vi "ramping waveform.vi"(6 "mode":u16(ring) items=["unidirection", "bidirection"], 8 "points in t2":dbl=500.0, 9 "points in t1":dbl=500.0, 10 "p2":dbl=10000.0, 11 "p1":dbl=10000.0) -> (3 "array":dbl[](array[numeric]))   [LabVIEW 2015]
panel:
  out "d":dbl=10000.0
  out "c":dbl=10000.0
  out "Waveform Graph":dbl[](graph)
  out "b":dbl=10000.0
  out "a":dbl=10000.0
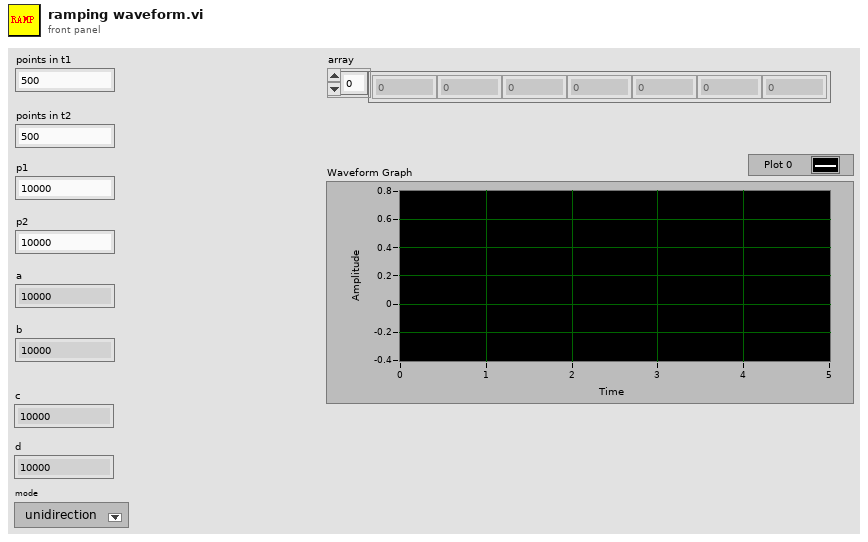
[diagram p1: front panel]
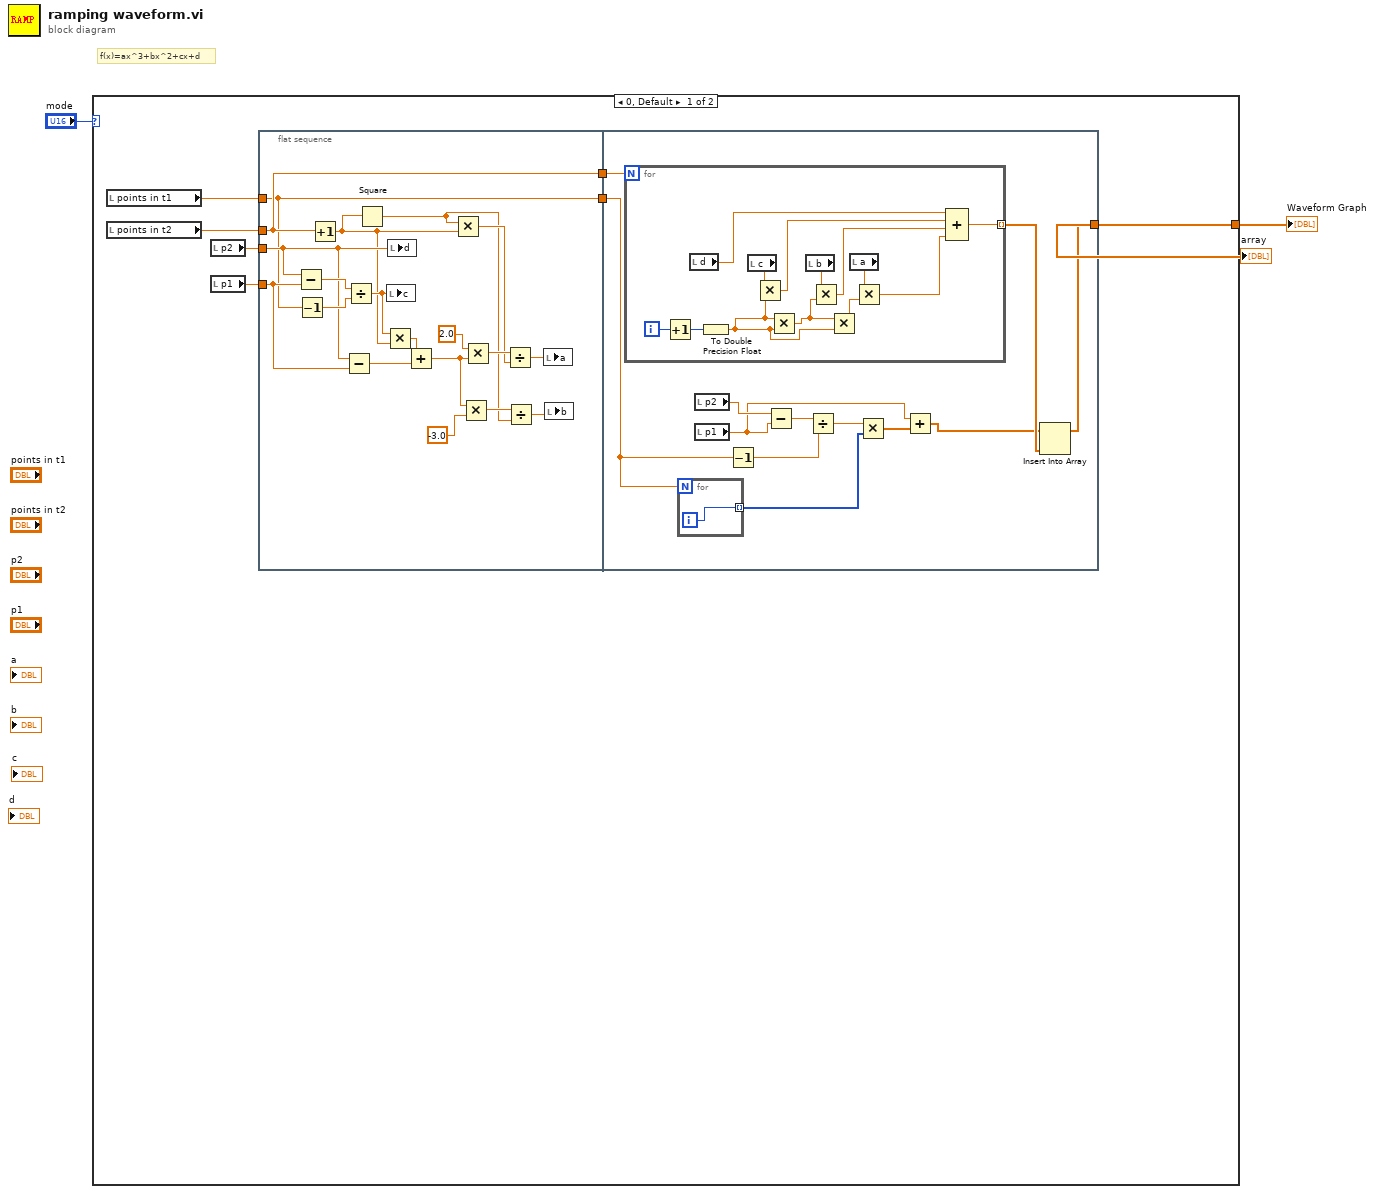
[diagram p0: block diagram]
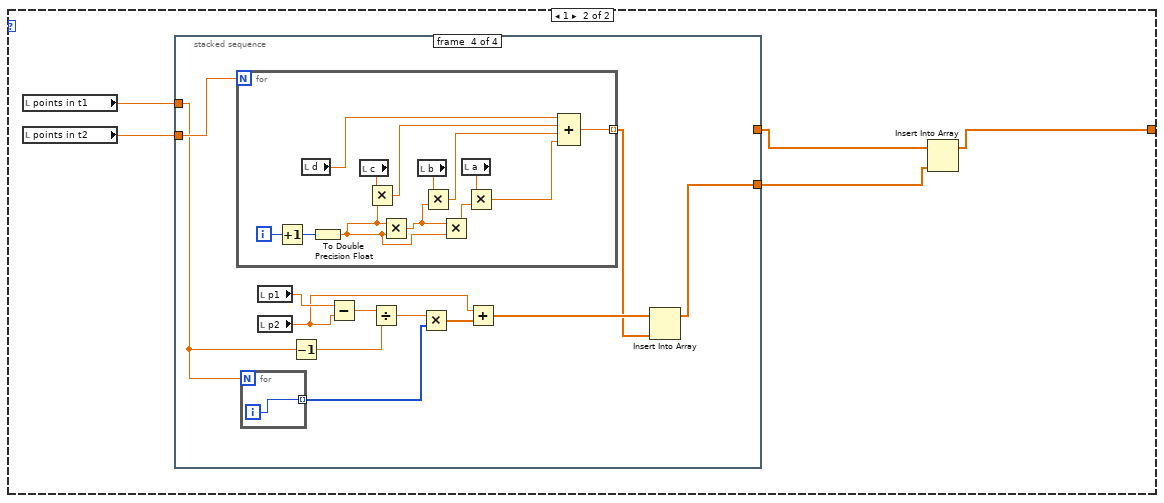
[diagram p2: hidden frame]
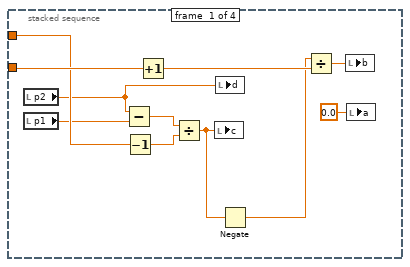
[diagram p3: hidden frame]
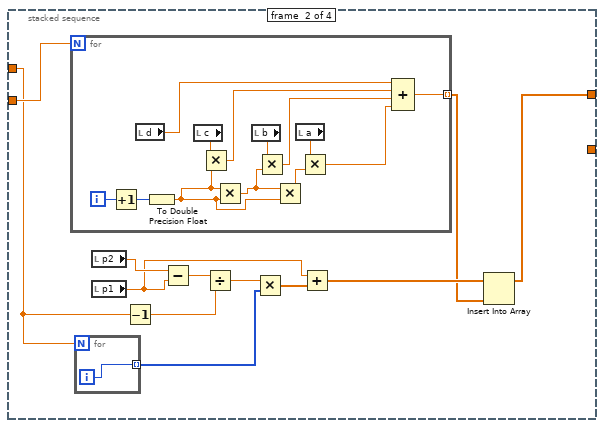
[diagram p4: hidden frame]
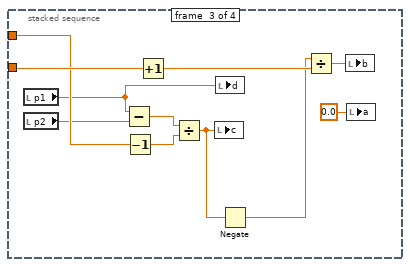
[diagram p5: hidden frame]
diagram:
  # "f(x)=ax^3+bx^2+cx+d"
  n1 = case shown="0, Default" "mode" {
    tunnel: [w9 w55] -> w1
    frame 0, Default {
      n2 = local read "points in t1"() -> (w5:dbl)
      n3 = local read "points in t2"() -> (w6:dbl)
      n4 = local read "p2"() -> (w7:dbl)
      n5 = local read "p1"() -> (w8:dbl)
      n6 = flat-sequence {
        tunnel: w6 -> [w24]
        tunnel: w7 -> [w23]
        tunnel: w8 -> [w22]
        tunnel: w5 -> [w10]
        tunnel: [w24] -> w4
        tunnel: [w10] -> w3
        tunnel: [w39] -> w9
        tunnel: w4 -> [w40]
        tunnel: w3 -> [w29]
        frame #0 {
          n7 = Subtract(x=w23, y=w22) -> (x-y=w28:dbl)
          n8 = Decrement(x=w10) -> (x-1=w27:dbl)
          n9 = Increment(x=w24) -> (x+1=w12:dbl)
          n10 = Subtract(x=w23, y=w22) -> (x-y=w20:dbl)
          n11 = Divide(x=w28, y=w27) -> (x/y=w25:dbl)
          n12 = Square(x=w12) -> (x^2=w11:dbl)
          n13 = Multiply(x=w25, y=w12) -> (x*y=w21:dbl)
          n14 = local write "c"(w25) -> ()
          n15 = local write "d"(w23) -> ()
          n16 = Add(x=w21, y=w20) -> (x+y=w16:dbl)
          n17 = Multiply(x=w11, y=w12) -> (x*y=w13:dbl)
          n18 = Multiply(x=w16, y=-3.0 ("x")) -> (x*y=w14:dbl)
          n19 = Multiply(x=2.0, y=w16) -> (x*y=w18:dbl)
          n20 = Divide(x=w18, y=w13) -> (x/y=w26:dbl)
          n21 = Divide(x=w14, y=w11) -> (x/y=w15:dbl)
          n22 = local write "a"(w26) -> ()
          n23 = local write "b"(w15) -> ()
        }
        frame #1 {
          n24 = for {
            N: w40 -> [_]
            tunnel: [w54] -> w38 mode=indexing
            i -> [w53]
            n25 = Increment(x=w53) -> (x+1=w52:i32)
            n26 = local read "d"() -> (w42:dbl)
            n27 = To Double Precision Float(number=w52) -> (double precision float=w47:dbl)
            n28 = local read "c"() -> (w46:dbl)
            n29 = Multiply(x=w46, y=w47) -> (x*y=w43:dbl)
            n30 = Multiply(x=w47, y=w47) -> (x*y=w48:dbl)
            n31 = local read "b"() -> (w49:dbl)
            n32 = Multiply(x=w49, y=w48) -> (x*y=w44:dbl)
            n33 = Multiply(x=w48, y=w47) -> (x*y=w51:dbl)
            n34 = local read "a"() -> (w50:dbl)
            n35 = Multiply(x=w50, y=w51) -> (x*y=w45:dbl)
            n36 = Compound Arithmetic op=ADD(w42, w43, w44, w45) -> (w54:dbl)
          }
          n37 = for {
            N: w29 -> [_]
            tunnel: [w41] -> w33 mode=indexing
            i -> [w41]
          }
          n38 = local read "p2"() -> (w37:dbl)
          n39 = local read "p1"() -> (w31:dbl)
          n40 = Decrement(x=w29) -> (x-1=w35:dbl)
          n41 = Subtract(x=w37, y=w31) -> (x-y=w36:dbl)
          n42 = Divide(x=w36, y=w35) -> (x/y=w34:dbl)
          n43 = Multiply(x=w34, y=w33) -> (x*y=w32:dbl[])
          n44 = Add(x=w31, y=w32) -> (x+y=w30:dbl[])
          n45 = Insert Into Array(array=w30, new element=w38) -> (w39:dbl[])  [unwired: 1 in]
        }
      }
    }
    frame 1 {
      n46 = local read "points in t1"() -> (w59:dbl)
      n47 = local read "points in t2"() -> (w58:dbl)
      n48 = stacked-sequence {
        tunnel: w58 -> [w68 w72 w105 w110]
        tunnel: w59 -> [w62 w71 w99 w109]
        tunnel: [_ w74 _ _] -> w57
        tunnel: [_ _ _ w108] -> w56
        frame #0 {
          n49 = local read "p2"() -> (w61:dbl)
          n50 = local read "p1"() -> (w60:dbl)
          n51 = Subtract(x=w61, y=w60) -> (x-y=w70:dbl)
          n52 = Decrement(x=w62) -> (x-1=w69:dbl)
          n53 = Increment(x=w68) -> (x+1=w66:dbl)
          n54 = Divide(x=w70, y=w69) -> (x/y=w65:dbl)
          n55 = local write "c"(w65) -> ()
          n56 = local write "d"(w61) -> ()
          n57 = Negate(x=w65) -> (-x=w64:dbl)
          n58 = Divide(x=w64, y=w66) -> (x/y=w67:dbl)
          n59 = local write "b"(w67) -> ()
          n60 = local write "a"(0.0 ("a")) -> ()
        }
        frame #1 {
          n61 = for {
            N: w72 -> [_]
            tunnel: [w96] -> w73 mode=indexing
            i -> [w95]
            n62 = Increment(x=w95) -> (x+1=w94:i32)
            n63 = local read "d"() -> (w84:dbl)
            n64 = To Double Precision Float(number=w94) -> (double precision float=w89:dbl)
            n65 = local read "c"() -> (w88:dbl)
            n66 = Multiply(x=w88, y=w89) -> (x*y=w85:dbl)
            n67 = Multiply(x=w89, y=w89) -> (x*y=w90:dbl)
            n68 = local read "b"() -> (w91:dbl)
            n69 = Multiply(x=w91, y=w90) -> (x*y=w86:dbl)
            n70 = Multiply(x=w90, y=w89) -> (x*y=w93:dbl)
            n71 = local read "a"() -> (w92:dbl)
            n72 = Multiply(x=w92, y=w93) -> (x*y=w87:dbl)
            n73 = Compound Arithmetic op=ADD(w84, w85, w86, w87) -> (w96:dbl)
          }
          n74 = for {
            N: w71 -> [_]
            tunnel: [w83] -> w78 mode=indexing
            i -> [w83]
          }
          n75 = local read "p2"() -> (w82:dbl)
          n76 = local read "p1"() -> (w76:dbl)
          n77 = Decrement(x=w71) -> (x-1=w80:dbl)
          n78 = Subtract(x=w82, y=w76) -> (x-y=w81:dbl)
          n79 = Divide(x=w81, y=w80) -> (x/y=w79:dbl)
          n80 = Multiply(x=w79, y=w78) -> (x*y=w77:dbl[])
          n81 = Add(x=w76, y=w77) -> (x+y=w75:dbl[])
          n82 = Insert Into Array(array=w75, new element=w73) -> (w74:dbl[])  [unwired: 1 in]
        }
        frame #2 {
          n83 = local read "p1"() -> (w98:dbl)
          n84 = local read "p2"() -> (w97:dbl)
          n85 = Subtract(x=w98, y=w97) -> (x-y=w107:dbl)
          n86 = Decrement(x=w99) -> (x-1=w106:dbl)
          n87 = Increment(x=w105) -> (x+1=w103:dbl)
          n88 = Divide(x=w107, y=w106) -> (x/y=w102:dbl)
          n89 = local write "c"(w102) -> ()
          n90 = local write "d"(w98) -> ()
          n91 = Negate(x=w102) -> (-x=w101:dbl)
          n92 = Divide(x=w101, y=w103) -> (x/y=w104:dbl)
          n93 = local write "b"(w104) -> ()
          n94 = local write "a"(0.0 ("a")) -> ()
        }
        frame #3 {
          n95 = for {
            N: w110 -> [_]
            tunnel: [w133] -> w111 mode=indexing
            i -> [w132]
            n96 = Increment(x=w132) -> (x+1=w131:i32)
            n97 = local read "d"() -> (w121:dbl)
            n98 = To Double Precision Float(number=w131) -> (double precision float=w126:dbl)
            n99 = local read "c"() -> (w125:dbl)
            n100 = Multiply(x=w125, y=w126) -> (x*y=w122:dbl)
            n101 = Multiply(x=w126, y=w126) -> (x*y=w127:dbl)
            n102 = local read "b"() -> (w128:dbl)
            n103 = Multiply(x=w128, y=w127) -> (x*y=w123:dbl)
            n104 = Multiply(x=w127, y=w126) -> (x*y=w130:dbl)
            n105 = local read "a"() -> (w129:dbl)
            n106 = Multiply(x=w129, y=w130) -> (x*y=w124:dbl)
            n107 = Compound Arithmetic op=ADD(w121, w122, w123, w124) -> (w133:dbl)
          }
          n108 = for {
            N: w109 -> [_]
            tunnel: [w120] -> w115 mode=indexing
            i -> [w120]
          }
          n109 = local read "p1"() -> (w119:dbl)
          n110 = local read "p2"() -> (w113:dbl)
          n111 = Decrement(x=w109) -> (x-1=w117:dbl)
          n112 = Subtract(x=w119, y=w113) -> (x-y=w118:dbl)
          n113 = Divide(x=w118, y=w117) -> (x/y=w116:dbl)
          n114 = Multiply(x=w116, y=w115) -> (x*y=w114:dbl[])
          n115 = Add(x=w113, y=w114) -> (x+y=w112:dbl[])
          n116 = Insert Into Array(array=w112, new element=w111) -> (w108:dbl[])  [unwired: 1 in]
        }
      }
      n117 = Insert Into Array(array=w57, new element=w56) -> (w55:dbl[])  [unwired: 1 in]
    }
  }
  "array" <- w1
  "Waveform Graph" <- w1
